vi "GetGearIntakeSpeed.vi"(11 "Gear Intake in":refnum<class "Gear Intake.lvclass">) -> (2 "Gear Intake Speed":dbl, 3 "Gear Intake out":refnum<class "Gear Intake.lvclass">)   [LabVIEW 2016, in "Gear Intake.lvclass"]
uses:
  Gear Intake.lvclass
  Gear Intake.lvclass/Gear Intake.ctl
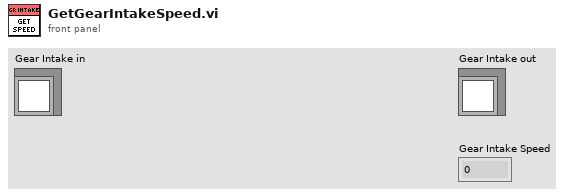
[diagram p1: front panel]
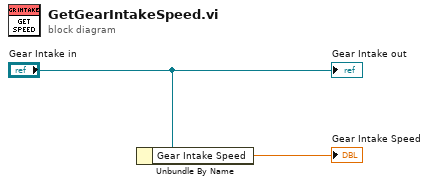
[diagram p0: block diagram]
diagram:
  n1 = Unbundle By Name("Gear Intake in") -> ("Gear Intake Speed"=→"Gear Intake Speed":dbl)
  "Gear Intake out" <- "Gear Intake in"
